vi "Filter (SubVI).vi"(9 "Delta":dbl=4000.0 format="%#_13g", 10 "NewVal":dbl, 11 "OldVal":dbl) -> (3 "Val":dbl)   [LabVIEW 2017]
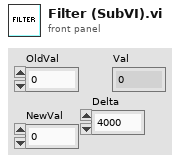
[diagram p1: front panel]
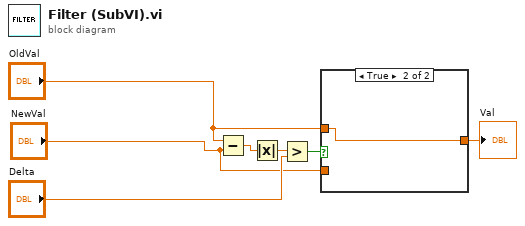
[diagram p0: block diagram]
diagram:
  n1 = Subtract(x="OldVal", y="NewVal") -> (x-y=w1:dbl)
  n2 = Absolute Value(x=w1) -> (abs(x)=w7:dbl)
  n3 = Greater?(x=w7, y="Delta") -> (0:w6:bool)
  n4 = case shown="True" w6 {
    tunnel: "OldVal" -> [_ w9]
    tunnel: "NewVal" -> [w8 _]
    tunnel: [w8 w9] -> w2
    frame False {
    }
    frame True {
    }
  }
  "Val" <- w2
